vi "Create 2D Data.vi"(1 "noise":dbl=0.003, 2 "Vsg":dbl[](array[numeric])=[0.089, 0.07933333333333334, 0.06966666666666667], 3 "width":dbl=0.003, 4 "dV":dbl=0.0001, 5 "NV":dbl=900.0, 6 "V0":dbl) -> (0 "XY Graph":cluster{dbl[], dbl[]}(graph))   [LabVIEW 2016]
uses:
  <vilib>/ptbypt/NI_PtbyPt.lvlib
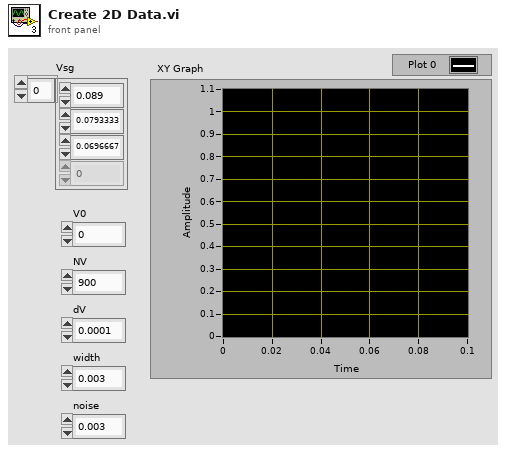
[diagram p1: front panel]
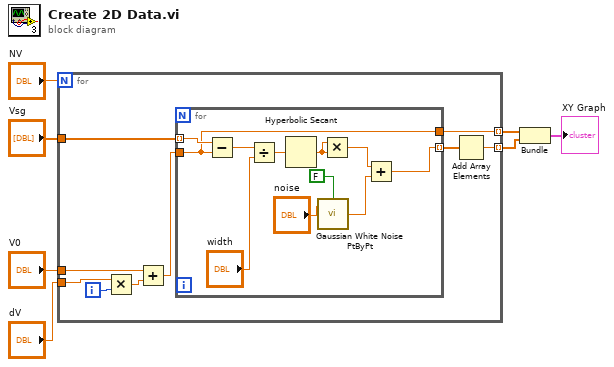
[diagram p0: block diagram]
diagram:
  n1 = for {
    N: "NV" -> [_]
    tunnel: "Vsg" -> [w16]
    tunnel: "V0" -> [w9]
    tunnel: "dV" -> [w10]
    tunnel: [w13] -> w4 mode=indexing
    tunnel: [w14] -> w3 mode=indexing
    i -> [w11]
    n2 = Multiply(x=w10, y=w11) -> (x*y=w12:dbl)
    n3 = Add(x=w9, y=w12) -> (x+y=w8:dbl)
    n4 = for {
      tunnel: w16 -> [w27] mode=indexing
      tunnel: [w17] -> w15 mode=indexing
      tunnel: [w25] -> w14
      tunnel: w8 -> [w25]
      n5 = Subtract(x=w27, y=w25) -> (x-y=w24:dbl)
      n6 = Divide(x=w24, y="width") -> (x/y=w22:dbl)
      n7 = Hyperbolic Secant(1:w22) -> (0:w26:dbl)
      n8 = call <vilib>:"Gaussian White Noise PtByPt.vi"("initialize"=FALSE, "standard deviation"="noise") -> ("Gaussian white noise"=w20:dbl)  [unwired: 1 in]
      n9 = Multiply(x=w26, y=w26) -> (x*y=w21:dbl)
      n10 = Add(x=w21, y=w20) -> (x+y=w17:dbl)
    }
    n11 = Add Array Elements(numeric array=w15) -> (sum=w13:dbl)
  }
  n12 = Bundle(w3, w4) -> (→"XY Graph":cluster{dbl[], dbl[]})  [unwired: 1 in]
